vi "PromVIEW Basic Metrics Example.vi"() -> ()   [LabVIEW 2020]
uses:
  src/metrics/gauge/Gauge.lvclass
  src/metrics/counter/Counter.lvclass
  src/registry/session/Registry Session.lvclass
panel:
  out "Timeout Values":i32(graph)
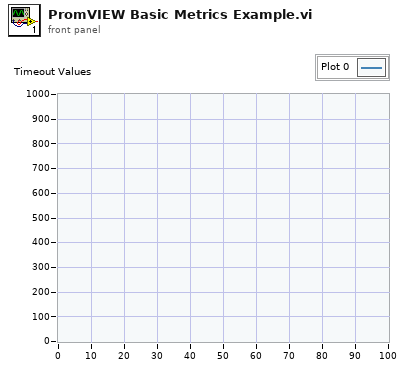
[diagram p1: front panel]
types:
  T1 = typedef "Registry.lvlib/Registry Session.lvclass/Session Handle.ctl" = refnum<data-value>
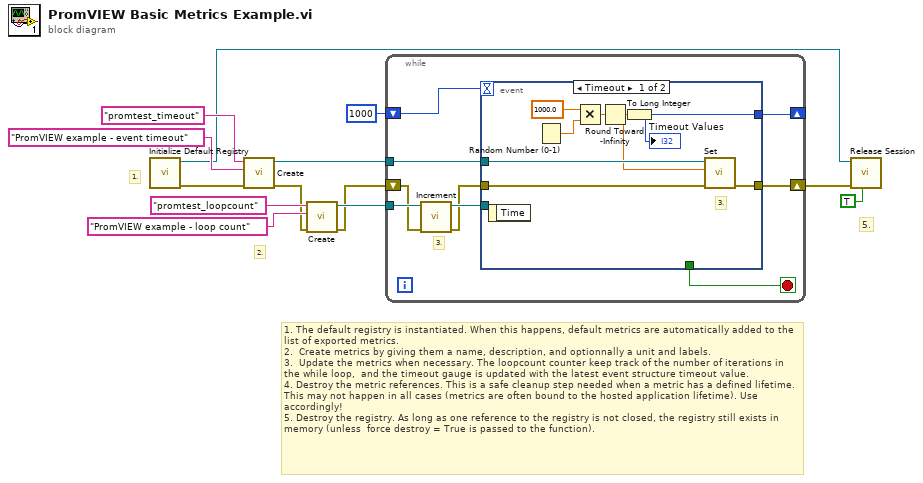
[diagram p0: block diagram]
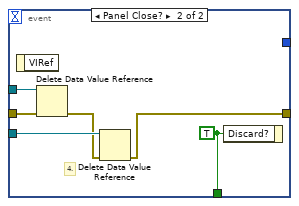
[diagram p2: hidden frame]
diagram:
  # "1. The default registry is instantiated. When this happens, default metrics are automatically added to the list of exported metrics.\n2.  Create metrics by giving them a name, description, and optionnally a unit and labels.\n3.  Update the metrics when necessary. The loopcount counter keep track of the number of iterations in the while loop,  and the timeout gauge is updated with the latest event structure timeout value.\n4. Destroy the metric references. This is a safe cleanup step needed when a metric has a defined lifetime. This may not happen in all cases (metrics are often bound to the hosted application lifetime). Use accordingly!\n5. Destroy the registry. As long as one reference to the registry is not closed, the registry still exists in memory (unless  force destroy = True is passed to the function)."
  # "5."
  # "2."
  # "1."
  n1 = call "Initialize Default Registry.vi"() -> ("error out"=w12:errorcluster, "Session Handle"=w5:T1)  [unwired: 9 in, 1 out]
  n2 = call "Create.vi"("error in (no error)"=w12, "Description"="PromVIEW example - event timeout", "Metric Name"="promtest_timeout") -> ("error out"=w2:errorcluster, "Gauge Ref"=w7:refnum<data-value>)  [unwired: 7 in]
  n3 = call "Create.vi"("error in (no error)"=w2, "Description"="PromVIEW example - loop count", "Metric Name"="promtest_loopcount") -> ("error out"=w1:errorcluster, "Counter Ref"=w6:refnum<data-value>)  [unwired: 7 in]
  n4 = while {
    shift-right: [w21] -> _
    shift-left: 1000 -> [w20]
    tunnel: w7 -> [w19]
    tunnel: w6 -> [w18]
    shift-right: [w17] -> w4
    shift-left: w1 -> [w15]
    stop <- w22 stop-if-true
    # "3."
    n5 = call "Increment.vi"("error in (no error)"=w15, "Counter Ref"=w18) -> ("error out"=w14:errorcluster, "Counter Ref out"=w16:refnum<data-value>)  [unwired: 8 in]
    n6 = event shown="[0] Timeout" {
      selector: _ -> [_ _]
      dyn-events: _ -> [_ _]
      timeout: w20 -> [_ _]
      tunnel: [_ w36] -> w22
      tunnel: [w24 _] -> w21
      tunnel: w19 -> [w27 w35]
      tunnel: w14 -> [w25 w33]
      tunnel: [w23 w31] -> w17
      tunnel: w16 -> [_ w34]
      event Timeout {
        # "3."
        n7 = event-data() -> ()  [unwired: 1 in, 1 out]
        n8 = Random Number (0-1)() -> (number: 0 to 1=w30:dbl)
        n9 = Multiply(x=1000.0, y=w30) -> (x*y=w28:dbl)
        n10 = Round Toward -Infinity(1:w28) -> (0:w26:dbl)
        n11 = To Long Integer(number=w26) -> (32bit integer=w24:i32)
        "Timeout Values" <- w24
        n12 = call "Set.vi"("error in (no error)"=w25, "Value"=w26, "Gauge Ref"=w27) -> ("error out"=w23:errorcluster)  [unwired: 7 in, 1 out]
      }
      event Panel Close? {
        w36 = TRUE ("Discard?")
        # "4."
        n13 = event-data() -> ()  [unwired: 1 in, 1 out]
        n14 = Delete Data Value Reference(data value reference=w35, error in=w33) -> (error out=w32:errorcluster)  [unwired: 1 out]
        n15 = Delete Data Value Reference(data value reference=w34, error in=w32) -> (error out=w31:errorcluster)  [unwired: 1 out]
        n16 = event-data("Discard?"=w36) -> ()  [unwired: 1 in, 1 out]
      }
    }
  }
  n17 = call "Release Session.vi"("force destroy? (F)"=TRUE, "error in (no error)"=w4, "Session Handle"=w5) -> ()  [unwired: 8 in, 1 out]
